vi "Controller List.vi"() -> (1 "Controller List":T2(array[cluster])=[{"Controller Name"=enum."Kuhnke", "CommSeg"=2, "PWM?"=TRUE, "Frequency"=100, "Low Command"=10.0, "High Command"=90.0, "Stop Command"=10.0, "Command Step"=0.1, "Solenoid Stop?"=FALSE, "Controller?"=TRUE, "Name"="Kuhnke", "Indirect Nonzero CMD"=15.0}, {"Controller Name"=enum."Helbako BLDC", "CommSeg"=2, "PWM?"=TRUE, "Frequency"=100, "Low Command"=10.0, "High Command"=90.0, "Stop Command"=10.0, "Command Step"=0.1, "Solenoid Stop?"=FALSE, "Controller?"=TRUE, "Name"="Helbako BLDC", "Indirect Nonzero CMD"=15.0}, {"Controller Name"=enum."Conti", "CommSeg"=2, "PWM?"=FALSE, "Frequency"=100, "Low Command"=0.0, "High Command"=800.0, "Stop Command"=0.0, "Command Step"=1.0, "Solenoid Stop?"=FALSE, "Controller?"=TRUE, "Name"="Conti", "Indirect Nonzero CMD"=0.0}, {"Controller Name"=enum."Hella BLDC Screw", "CommSeg"=2, "PWM?"=FALSE, "Frequency"=100, "Low Command"=0.0, "High Command"=100.0, "Stop Command"=0.0, "Command Step"=1.0, "Solenoid Stop?"=FALSE, "Controller?"=TRUE, "Name"="Hella BLDC Screw", "Indirect Nonzero CMD"=10.0}, {"Controller Name"=enum."Hella BLDC Turbine", "CommSeg"=2, "PWM?"=FALSE, "Frequency"=100, "Low Command"=0.0, "High Command"=100.0, "Stop Command"=0.0, "Command Step"=1.0, "Solenoid Stop?"=FALSE, "Controller?"=TRUE, "Name"="Hella BLDC Turbine", "Indirect Nonzero CMD"=10.0}, {"Controller Name"=enum."Helbako (old)", "CommSeg"=2, "PWM?"=FALSE, "Frequency"=100, "Low Command"=0.0, "High Command"=100.0, "Stop Command"=0.0, "Command Step"=0.1, "Solenoid Stop?"=FALSE, "Controller?"=TRUE, "Name"="Helbako (old)", "Indirect Nonzero CMD"=0.0}, {"Controller Name"=enum."TI PWM", "CommSeg"=2, "PWM?"=TRUE, "Frequency"=100, "Low Command"=0.0, "High Command"=100.0, "Stop Command"=0.0, "Command Step"=0.1, "Solenoid Stop?"=FALSE, "Controller?"=TRUE, "Name"="TI PWM", "Indirect Nonzero CMD"=0.0}, {"Controller Name"=enum."PSA", "CommSeg"=2, "PWM?"=TRUE, "Frequency"=100, "Low Command"=5.0, "High Command"=95.0, "Stop Command"=5.0, "Command Step"=0.1, "Solenoid Stop?"=FALSE, "Controller?"=TRUE, "Name"="PSA", "Indirect Nonzero CMD"=5.0}, {"Controller Name"=enum."Hella Gas", "CommSeg"=2, "PWM?"=FALSE, "Frequency"=100, "Low Command"=0.0, "High Command"=800.0, "Stop Command"=0.0, "Command Step"=1.0, "Solenoid Stop?"=TRUE, "Controller?"=TRUE, "Name"="Hella Gas", "Indirect Nonzero CMD"=0.0}, {"Controller Name"=enum."Hella Diesel", "CommSeg"=10, "PWM?"=FALSE, "Frequency"=100, "Low Command"=370.0, "High Command"=461.0, "Stop Command"=370.0, "Command Step"=1.0, "Solenoid Stop?"=TRUE, "Controller?"=TRUE, "Name"="Hella Diesel", "Indirect Nonzero CMD"=370.0}, {"Controller Name"=enum."8 Comm", "CommSeg"=8, "PWM?"=FALSE, "Frequency"=150, "Low Command"=0.0, "High Command"=1.0, "Stop Command"=0.0, "Command Step"=1.0, "Solenoid Stop?"=FALSE, "Controller?"=FALSE, "Name"="8 Comm", "Indirect Nonzero CMD"=0.0}, {"Controller Name"=enum."10 Comm", "CommSeg"=10, "PWM?"=FALSE, "Frequency"=150, "Low Command"=0.0, "High Command"=1.0, "Stop Command"=0.0, "Command Step"=1.0, "Solenoid Stop?"=FALSE, "Controller?"=FALSE, "Name"="10 Comm", "Indirect Nonzero CMD"=0.0}, {"Controller Name"=enum."8 Comm Hella", "CommSeg"=8, "PWM?"=TRUE, "Frequency"=150, "Low Command"=0.0, "High Command"=50.0, "Stop Command"=80.0, "Command Step"=0.1, "Solenoid Stop?"=FALSE, "Controller?"=TRUE, "Name"="8 Comm Hella", "Indirect Nonzero CMD"=0.0}, {"Controller Name"=enum."10 Comm Hella", "CommSeg"=10, "PWM?"=TRUE, "Frequency"=150, "Low Command"=0.0, "High Command"=50.0, "Stop Command"=80.0, "Command Step"=0.1, "Solenoid Stop?"=FALSE, "Controller?"=TRUE, "Name"="10 Comm Hella", "Indirect Nonzero CMD"=0.0}, {"Controller Name"=enum."8 Comm Omron", "CommSeg"=8, "PWM?"=TRUE, "Frequency"=150, "Low Command"=5.0, "High Command"=50.0, "Stop Command"=75.0, "Command Step"=0.1, "Solenoid Stop?"=FALSE, "Controller?"=TRUE, "Name"="8 Comm Omron", "Indirect Nonzero CMD"=5.0}, {"Controller Name"=enum."10 Comm Omron", "CommSeg"=10, "PWM?"=TRUE, "Frequency"=150, "Low Command"=5.0, "High Command"=50.0, "Stop Command"=75.0, "Command Step"=0.1, "Solenoid Stop?"=FALSE, "Controller?"=TRUE, "Name"="10 Comm Omron", "Indirect Nonzero CMD"=5.0}, {"Controller Name"=enum."8 Comm Nissan", "CommSeg"=8, "PWM?"=TRUE, "Frequency"=10, "Low Command"=50.0, "High Command"=90.0, "Stop Command"=50.0, "Command Step"=0.1, "Solenoid Stop?"=TRUE, "Controller?"=TRUE, "Name"="8 Comm Nissan", "Indirect Nonzero CMD"=50.0}, {"Controller Name"=enum."10 Comm Nissan", "CommSeg"=10, "PWM?"=TRUE, "Frequency"=10, "Low Command"=50.0, "High Command"=90.0, "Stop Command"=50.0, "Command Step"=0.1, "Solenoid Stop?"=TRUE, "Controller?"=TRUE, "Name"="10 Comm Nissan", "Indirect Nonzero CMD"=50.0}])   [LabVIEW 2013]
uses:
  Controller Names.ctl
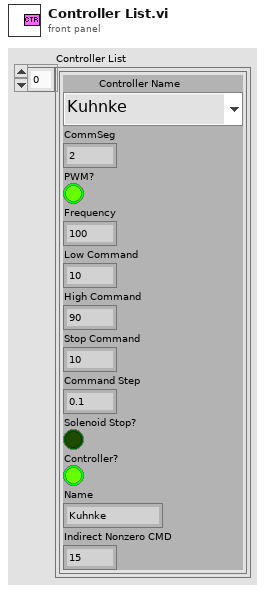
[diagram p1: front panel]
types:
  T1 = typedef "Controller Names.ctl" = enum16{"Kuhnke", "Helbako BLDC", "Conti", "Hella BLDC Screw", "Hella BLDC Turbine", "Helbako (old)", "TI PWM", "PSA", "Hella Gas", "Hella Diesel", "8 Comm", "10 Comm", "8 Comm Hella", "10 Comm Hella", "8 Comm Omron", "10 Comm Omron", "8 Comm Nissan", "10 Comm Nissan"}
  T2 = cluster{"Controller Name":T1, "CommSeg":i32, "PWM?":bool, "Frequency":i32, "Low Command":dbl, "High Command":dbl, "Stop Command":dbl, "Command Step":dbl, "Solenoid Stop?":bool, "Controller?":bool, "Name":string, "Indirect Nonzero CMD":dbl}[]
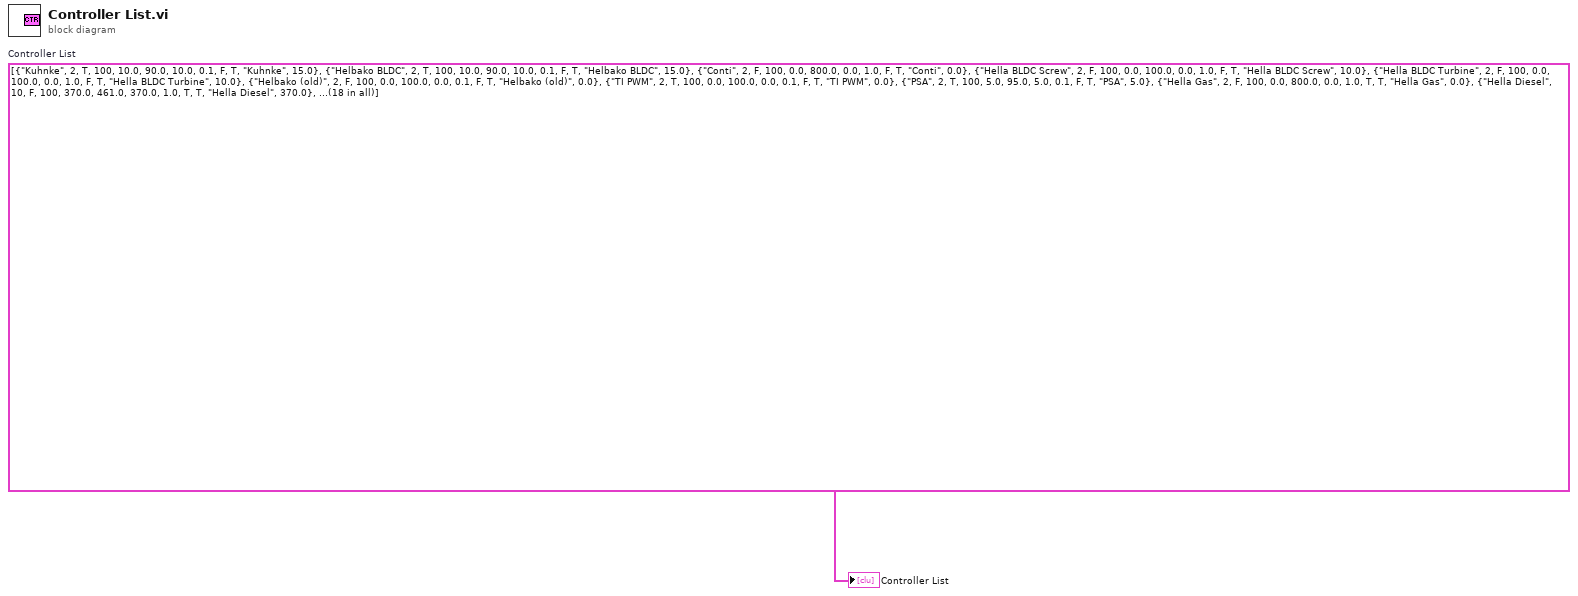
[diagram p0: block diagram]
diagram:
  w1 = T2 [{"Controller Name"=enum."Kuhnke", "CommSeg"=2, "PWM?"=TRUE, "Frequency"=100, "Low Command"=10.0, "High Command"=90.0, "Stop Command"=10.0, "Command Step"=0.1, "Solenoid Stop?"=FALSE, "Controller?"=TRUE, "Name"="Kuhnke", "Indirect Nonzero CMD"=15.0}, {"Controller Name"=enum."Helbako BLDC", "CommSeg"=2, "PWM?"=TRUE, "Frequency"=100, "Low Command"=10.0, "High Command"=90.0, "Stop Command"=10.0, "Command Step"=0.1, "Solenoid Stop?"=FALSE, "Controller?"=TRUE, "Name"="Helbako BLDC", "Indirect Nonzero CMD"=15.0}, {"Controller Name"=enum."Conti", "CommSeg"=2, "PWM?"=FALSE, "Frequency"=100, "Low Command"=0.0, "High Command"=800.0, "Stop Command"=0.0, "Command Step"=1.0, "Solenoid Stop?"=FALSE, "Controller?"=TRUE, "Name"="Conti", "Indirect Nonzero CMD"=0.0}, {"Controller Name"=enum."Hella BLDC Screw", "CommSeg"=2, "PWM?"=FALSE, "Frequency"=100, "Low Command"=0.0, "High Command"=100.0, "Stop Command"=0.0, "Command Step"=1.0, "Solenoid Stop?"=FALSE, "Controller?"=TRUE, "Name"="Hella BLDC Screw", "Indirect Nonzero CMD"=10.0}, {"Controller Name"=enum."Hella BLDC Turbine", "CommSeg"=2, "PWM?"=FALSE, "Frequency"=100, "Low Command"=0.0, "High Command"=100.0, "Stop Command"=0.0, "Command Step"=1.0, "Solenoid Stop?"=FALSE, "Controller?"=TRUE, "Name"="Hella BLDC Turbine", "Indirect Nonzero CMD"=10.0}, {"Controller Name"=enum."Helbako (old)", "CommSeg"=2, "PWM?"=FALSE, "Frequency"=100, "Low Command"=0.0, "High Command"=100.0, "Stop Command"=0.0, "Command Step"=0.1, "Solenoid Stop?"=FALSE, "Controller?"=TRUE, "Name"="Helbako (old)", "Indirect Nonzero CMD"=0.0}, {"Controller Name"=enum."TI PWM", "CommSeg"=2, "PWM?"=TRUE, "Frequency"=100, "Low Command"=0.0, "High Command"=100.0, "Stop Command"=0.0, "Command Step"=0.1, "Solenoid Stop?"=FALSE, "Controller?"=TRUE, "Name"="TI PWM", "Indirect Nonzero CMD"=0.0}, {"Controller Name"=enum."PSA", "CommSeg"=2, "PWM?"=TRUE, "Frequency"=100, "Low Command"=5.0, "High Command"=95.0, "Stop Command"=5.0, "Command Step"=0.1, "Solenoid Stop?"=FALSE, "Controller?"=TRUE, "Name"="PSA", "Indirect Nonzero CMD"=5.0}, {"Controller Name"=enum."Hella Gas", "CommSeg"=2, "PWM?"=FALSE, "Frequency"=100, "Low Command"=0.0, "High Command"=800.0, "Stop Command"=0.0, "Command Step"=1.0, "Solenoid Stop?"=TRUE, "Controller?"=TRUE, "Name"="Hella Gas", "Indirect Nonzero CMD"=0.0}, {"Controller Name"=enum."Hella Diesel", "CommSeg"=10, "PWM?"=FALSE, "Frequency"=100, "Low Command"=370.0, "High Command"=461.0, "Stop Command"=370.0, "Command Step"=1.0, "Solenoid Stop?"=TRUE, "Controller?"=TRUE, "Name"="Hella Diesel", "Indirect Nonzero CMD"=370.0}, {"Controller Name"=enum."8 Comm", "CommSeg"=8, "PWM?"=FALSE, "Frequency"=150, "Low Command"=0.0, "High Command"=1.0, "Stop Command"=0.0, "Command Step"=1.0, "Solenoid Stop?"=FALSE, "Controller?"=FALSE, "Name"="8 Comm", "Indirect Nonzero CMD"=0.0}, {"Controller Name"=enum."10 Comm", "CommSeg"=10, "PWM?"=FALSE, "Frequency"=150, "Low Command"=0.0, "High Command"=1.0, "Stop Command"=0.0, "Command Step"=1.0, "Solenoid Stop?"=FALSE, "Controller?"=FALSE, "Name"="10 Comm", "Indirect Nonzero CMD"=0.0}, {"Controller Name"=enum."8 Comm Hella", "CommSeg"=8, "PWM?"=TRUE, "Frequency"=150, "Low Command"=0.0, "High Command"=50.0, "Stop Command"=80.0, "Command Step"=0.1, "Solenoid Stop?"=FALSE, "Controller?"=TRUE, "Name"="8 Comm Hella", "Indirect Nonzero CMD"=0.0}, {"Controller Name"=enum."10 Comm Hella", "CommSeg"=10, "PWM?"=TRUE, "Frequency"=150, "Low Command"=0.0, "High Command"=50.0, "Stop Command"=80.0, "Command Step"=0.1, "Solenoid Stop?"=FALSE, "Controller?"=TRUE, "Name"="10 Comm Hella", "Indirect Nonzero CMD"=0.0}, {"Controller Name"=enum."8 Comm Omron", "CommSeg"=8, "PWM?"=TRUE, "Frequency"=150, "Low Command"=5.0, "High Command"=50.0, "Stop Command"=75.0, "Command Step"=0.1, "Solenoid Stop?"=FALSE, "Controller?"=TRUE, "Name"="8 Comm Omron", "Indirect Nonzero CMD"=5.0}, {"Controller Name"=enum."10 Comm Omron", "CommSeg"=10, "PWM?"=TRUE, "Frequency"=150, "Low Command"=5.0, "High Command"=50.0, "Stop Command"=75.0, "Command Step"=0.1, "Solenoid Stop?"=FALSE, "Controller?"=TRUE, "Name"="10 Comm Omron", "Indirect Nonzero CMD"=5.0}, {"Controller Name"=enum."8 Comm Nissan", "CommSeg"=8, "PWM?"=TRUE, "Frequency"=10, "Low Command"=50.0, "High Command"=90.0, "Stop Command"=50.0, "Command Step"=0.1, "Solenoid Stop?"=TRUE, "Controller?"=TRUE, "Name"="8 Comm Nissan", "Indirect Nonzero CMD"=50.0}, {"Controller Name"=enum."10 Comm Nissan", "CommSeg"=10, "PWM?"=TRUE, "Frequency"=10, "Low Command"=50.0, "High Command"=90.0, "Stop Command"=50.0, "Command Step"=0.1, "Solenoid Stop?"=TRUE, "Controller?"=TRUE, "Name"="10 Comm Nissan", "Indirect Nonzero CMD"=50.0}]  # Controller List
  "Controller List" <- w1
